vi "S2DS_ClearPlot.vi"(2 "Clear plot?":bool, 3 "Cluster in":T1) -> (1 "Cluster out":T1)   [LabVIEW 2025]
uses:
  TYPE DEFS/S2DS_PlotInfo.ctl
  TYPE DEFS/S2DS_PlotCluster.ctl
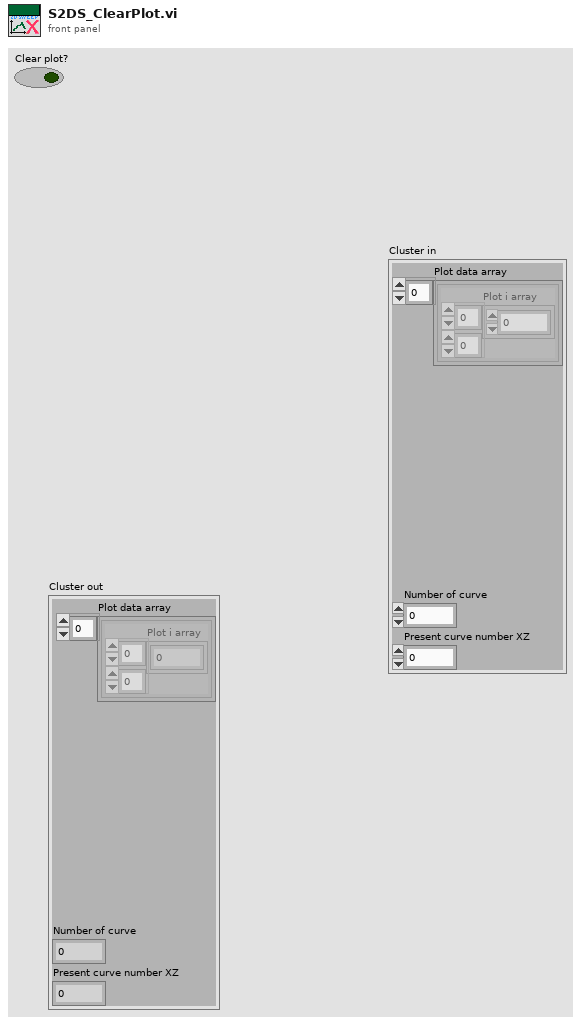
[diagram p1: front panel]
types:
  T1 = typedef "S2DS_PlotInfo.ctl" = cluster{"Plot data array":T2, "Number of curve":i32, "Present curve number XZ":i32}
  T2 = typedef "S2DS_PlotCluster.ctl" = cluster{"Plot i array":dbl[][]}[]
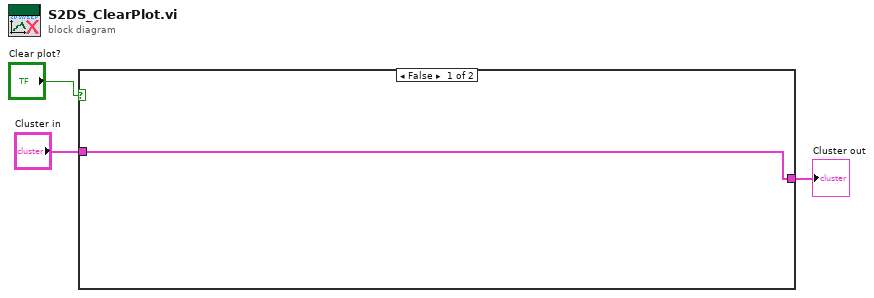
[diagram p0: block diagram]
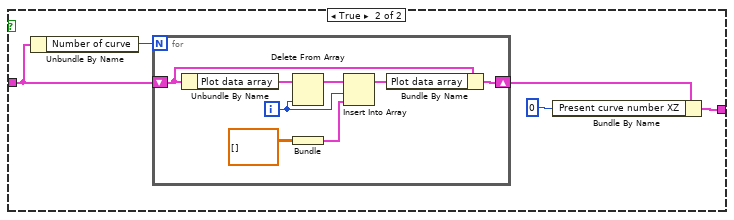
[diagram p2: hidden frame]
diagram:
  n1 = case shown="False" "Clear plot?" {
    tunnel: "Cluster in" -> [w4 w9]
    tunnel: [w4 w7] -> w1
    frame False {
    }
    frame True {
      n2 = Unbundle By Name(w9) -> ("Number of curve"=w8:i32)
      n3 = for {
        N: w8 -> [_]
        shift-right: [w14] -> w5
        shift-left: w9 -> [w15]
        i -> [w16]
        n4 = Unbundle By Name(w15) -> ("Plot data array"=w17:T2)
        n5 = Delete From Array(array=w17, index=w16) -> (array with subset deleted=w12:T2)  [unwired: 1 in, 1 out]
        n6 = Bundle(dbl[][] []) -> (w10:cluster{dbl[][]})  [unwired: 1 in]
        n7 = Insert Into Array(array=w12, index=w16, new element=w10) -> (w13:T2)
        n8 = Bundle By Name(cluster=w15, "Plot data array"=w13) -> (w14:T1)
      }
      n9 = Bundle By Name(cluster=w5, "Present curve number XZ"=0) -> (w7:T1)
    }
  }
  "Cluster out" <- w1
